vi "TransformTo360_171213.vi"(10 "nextY":dbl, 11 "nextX":dbl) -> (2 "X":i32, 3 "Y":i32)   [LabVIEW 2016]
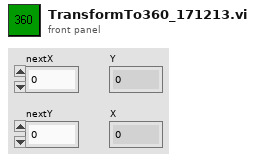
[diagram p1: front panel]
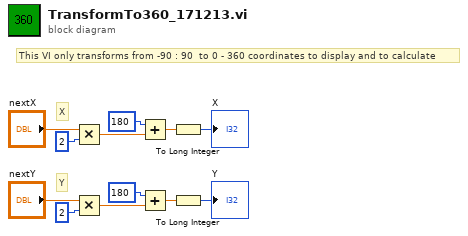
[diagram p0: block diagram]
diagram:
  # "This VI only transforms from -90 : 90  to 0 - 360 coordinates to display and to calculate"
  # "Y"
  # "X"
  n1 = Multiply(x="nextX", y=2 ("disabled index (col)")) -> (x*y=w5:dbl)
  n2 = Multiply(x="nextY", y=2 ("disabled index (col)")) -> (x*y=w6:dbl)
  n3 = Add(x=180 ("disabled index (col)"), y=w5) -> (x+y=w12:dbl)
  n4 = Add(x=180 ("disabled index (col)"), y=w6) -> (x+y=w11:dbl)
  n5 = To Long Integer(number=w12) -> (32bit integer=→"X":i32)
  n6 = To Long Integer(number=w11) -> (32bit integer=→"Y":i32)
